vi "FPGA_8a_ws_BIdireccional.vi"() -> ()   [LabVIEW 2015]
doc: "This VI reads a buffer of single point values from all four channels of the NI 923x and places the acquired data into a DMA FIFO."
uses:
  <vilib>/LabVIEW Targets/FPGA/cRIO/shared/nicrio_ModuleControls/nicrio_cRIO-9234_DataRatesRing2.ctl
  <vilib>/LabVIEW Targets/FPGA/cRIO/shared/nicrio_ModuleControls/nicrio_BasicConversionTime.ctl
  <vilib>/rvi/Emulation/niFpgaGetClockAttributes.vi
  <vilib>/rvi/Emulation/niFpgaSctlEmulationGetInTimedLoop.vi
  <vilib>/rvi/Emulation/niFpgaEmulationReportErrorSimple.vi
  <vilib>/rvi/eio/common/nirviEmuTemplateMethod_errors.vi
  <vilib>/rvi/Emulation/niFpgaCriticalErrorInLSC.vi
  <vilib>/rvi/eio/common/nirviEmuTemplatePropertySet_errors.vi
  <vilib>/rvi/Emulation/niFpgaProcessEmulError.vi
  <vilib>/rvi/interface/RandomDataEmulation/niFpgaRandomDataHandleErrors.vi
  <vilib>/eio/EIONode/EIONode.xnode
  <vilib>/eio/EIOPropertyNode/EIOPropertyNode.xnode
  <vilib>/rvi/DataTransferAndStorage/Container/XNode/niFpgaContainer.xnode
  <vilib>/rvi/interface/RandomDataEmulation/nirviRandomDataFpgaReadWriteTemplate.vi
  <vilib>/rvi/eio/common/nirviEmuTemplatePropertyGet_errors.vi
  <vilib>/rvi/eio/common/nirviEmuTemplatePropertyGet_noerrors.vi
  <vilib>/rvi/eio/common/nirviEmuTemplatePropertySet_noerrors.vi
panel:
  out "Direccion 0?":bool
  in  "Digital?":bool=TRUE
  out "Numeric 2":i32
  out "WhlCnt":fxp<+/-,24,-4> format="%.27g"
  in  "Offset_rueda":fxp<+/-,24,-4> format="%.27g"
  out "Rueda?":i16
  in  "Conversion Time":T1
  in  "Canal ccero?":bool=TRUE
  in  "Count(mSec)":u32=2
  out "Chassis Temperature":i16
  out "Fotocelula":bool
  out "Detector de\npresencia":bool
  in  "Fotocélula":bool
  out "DC OK":bool
  in  "Data Rate":T2=2 items=["51.200 kS/s (NI 9234)"=1, "25.600 kS/s (NI 9234)"=2, "17.067 kS/s (NI 9234)"=3, "12.800 kS/s (NI 9234)"=4, "10.240 kS/s (NI 9234)"=5, "8.533 kS/s (NI 9234)"=6, "7.314 kS/s (NI 9234)"=7, "6.400 kS/s (NI 9234)"=8, "5.689 kS/s (NI 9234)"=9, "5.120 kS/s (NI 9234)"=10, "4.654 kS/s (NI 9234)"=11, "4.267 kS/s (NI 9234)"=12, "3.938 kS/s (NI 9234)"=13, "3.657 kS/s (NI 9234)"=14, "3.413 kS/s (NI 9234)"=15, "3.200 kS/s (NI 9234)"=16, "3.012 kS/s (NI 9234)"=17, "2.845 kS/s (NI 9234)"=18, "2.695 kS/s (NI 9234)"=19, "2.560 kS/s (NI 9234)"=20, "2.438 kS/s (NI 9234)"=21, "2.328 kS/s (NI 9234)"=22, "2.226 kS/s (NI 9234)"=23, "2.133 kS/s (NI 9234)"=24, "2.048 kS/s (NI 9234)"=25, "1.969 kS/s (NI 9234)"=26, "1.896 kS/s (NI 9234)"=27, "1.829 kS/s (NI 9234)"=28, "1.765 kS/s (NI 9234)"=29, "1.707 kS/s (NI 9234)"=30, "1.652 kS/s (NI 9234)"=31]
  out "Buffer Overflow":bool
  in  "Stop":bool
  out "Buffer Underflow":bool
  out "Error Out":errorcluster
  # "For instructions, and select Help>>Show Context Help and hover over the icon."
  # "Timing Parameters"
  # "Output Parameters"
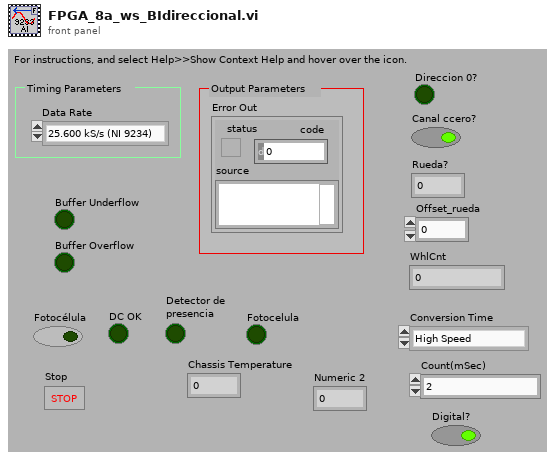
[diagram p1: front panel]
types:
  T1 = typedef "nicrio_BasicConversionTime.ctl" = enum8{"High Speed", "High Resolution"}
  T2 = typedef "nicrio_cRIO-9234_DataRatesRing2.ctl" = u8
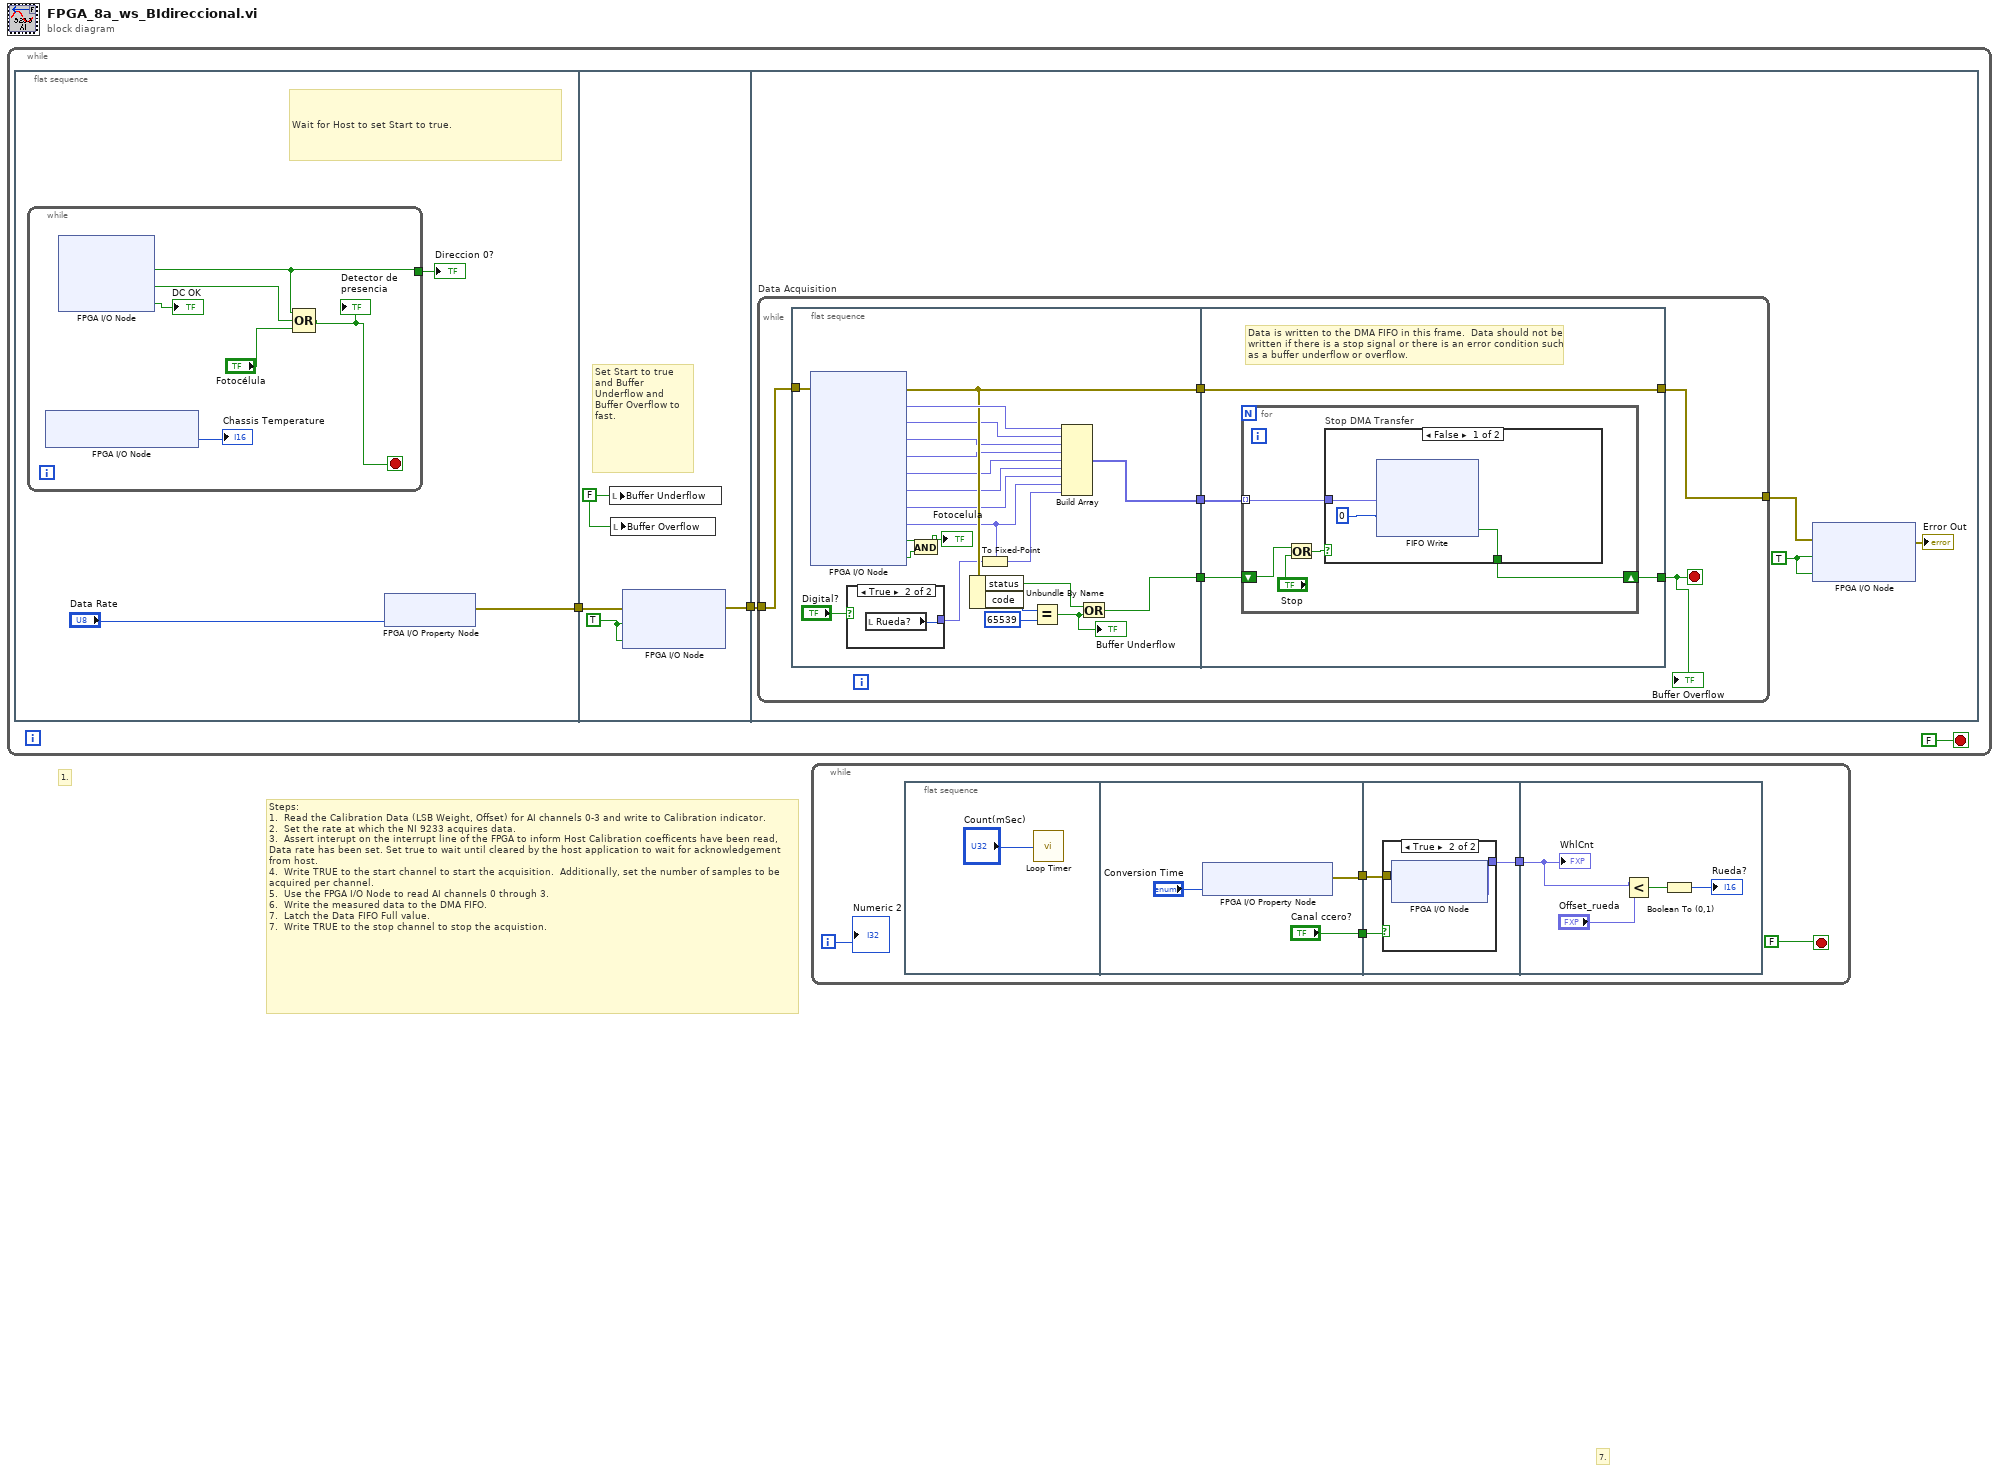
[diagram p0: block diagram]
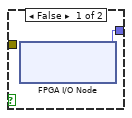
[diagram p2: hidden frame]
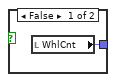
[diagram p3: hidden frame]
diagram:
  # "7."
  # "Steps: \n1.  Read the Calibration Data (LSB Weight, Offset) for AI channels 0-3 and write to Calibration indicator.\n2.  Set the rate at which the NI 9233 acquires data. \n3.  Assert interupt on the interrupt line of the FPGA to inform Host Calibration coefficents have been read, Data rate has been set. Set true to wait until cleared by the host application to wait for acknowledgement from host.\n4.  Write TRUE to the start channel to start the acquisition.  Additionally, set the number of samples to be acquired per channel.\n5.  Use the FPGA I/O Node to read AI channels 0 through 3. \n6.  Write the measured data to the DMA FIFO.\n7.  Latch the Data FIFO Full value.\n7.  Write TRUE to the stop channel to stop the acquistion."
  # "1."
  n1 = while {
    stop <- FALSE stop-if-true
    n2 = flat-sequence "MainSeq" {
      tunnel: [w6] -> w2
      tunnel: w2 -> [w15]
      tunnel: [w14] -> w1
      tunnel: w1 -> [w20]
      frame #0 {
        # "Wait for Host to set Start to true."
        n3 = while "initWait" {
          tunnel: [w7] -> w4
          stop <- w8 stop-if-true
          n4 = xnode "FPGA I/O Node"() -> ("Chassis Temperature"=→"Chassis Temperature":i16)  [unwired: 1 in, 1 out]
          n5 = xnode "FPGA I/O Node"() -> ("Mod3/DI0"=w7:bool, "Mod3/DI1"=w10:bool, "Mod3/DI2"=→"DC OK":bool)  [unwired: 4 in, 4 out]
          n6 = Compound Arithmetic op=OR(w7, w10, "Fotocélula") -> (w8:bool)
          "Detector de\npresencia" <- w8
        }
        "Direccion 0?" <- w4
        n7 = xnode "FPGA I/O Property Node"("Data Rate"="Data Rate") -> ("error out"=w6:errorcluster)  [unwired: 2 in, 1 out]
      }
      frame #1 {
        w13 = TRUE
        w16 = FALSE ("Late? (Latched)")
        # "Set Start to true and Buffer Underflow and Buffer Overflow to fast."
        n8 = local write "Buffer Underflow"(w16) -> ()
        n9 = local write "Buffer Overflow"(w16) -> ()
        n10 = xnode "FPGA I/O Node"("error in"=w15, "Mod1/Start"=w13, "Mod2/Start"=w13) -> ("error out"=w14:errorcluster)  [unwired: 2 in, 2 out]
      }
      frame #2 {
        w17 = TRUE
        n11 = while "Data Acquisition" {
          tunnel: w20 -> [w24]
          tunnel: [w23] -> w18
          stop <- w21 stop-if-true
          n12 = flat-sequence "Data Acquisition Sequence" {
            tunnel: [w47] -> w26
            tunnel: [w38] -> w25
            tunnel: w24 -> [w46]
            tunnel: [w45] -> w22
            tunnel: w26 -> [w54]
            tunnel: w25 -> [w53]
            tunnel: [w52] -> w21
            tunnel: [w51] -> w23
            tunnel: w22 -> [w51]
            frame #0 {
              n13 = xnode "FPGA I/O Node"("error in"=w46) -> ("error out"=w45:errorcluster, "Mod1/AI0"=w48:fxp<+/-,24,4>, "Mod1/AI1"=w41:fxp<+/-,24,4>, "Mod1/AI2"=w40:fxp<+/-,24,4>, "Mod1/AI3"=w39:fxp<+/-,24,4>, "Mod2/AI0"=w36:fxp<+/-,24,4>, "Mod2/AI1"=w35:fxp<+/-,24,4>, "Mod2/AI2"=w34:fxp<+/-,24,4>, "Mod2/AI3"=w33:fxp<+/-,24,4>, "Mod3/DI0"=w29:bool, "Mod3/DI1"=w28:bool)  [unwired: 10 in, 10 out]
              n14 = case shown="True" "Digital?" {
                tunnel: [w49 w50] -> w30
                frame False {
                  n15 = local read "WhlCnt"() -> (w49:fxp<+/-,24,-4>)
                }
                frame True {
                  n16 = local read "Rueda?"() -> (w50:i16)
                }
              }
              n17 = And(x=w29, y=w28) -> (x .and. y?=→"Fotocelula":bool)
              n18 = Unbundle By Name(w45) -> ("status"=w37:bool, "code"=w44:i32)
              n19 = To Fixed-Point(fixed-point type=w33, number=w30) -> (fixed-point=w32:fxp<+/-,24,4>)
              n20 = Equal?(x=w44, y=65539) -> (x = y?=w42:bool)
              "Buffer Underflow" <- w42
              n21 = Build Array(w48, w41, w40, w39, w36, w35, w34, w33, w32) -> (w47:fxp<+/-,24,4>[])
              n22 = Or(x=w37, y=w42) -> (x .or. y?=w38:bool)
            }
            frame #1 {
              # "Data is written to the DMA FIFO in this frame.  Data should not be\nwritten if there is a stop signal or there is an error condition such \nas a buffer underflow or overflow."
              n23 = for "DMAWriteLoop" {
                tunnel: w54 -> [w59] mode=indexing
                shift-right: [w55] -> w52
                shift-left: w53 -> [w57]
                n24 = Or(x=w57, y="Stop") -> (x .or. y?=w56:bool)
                n25 = case "Stop DMA Transfer" shown="False" w56 {
                  selector: w56 -> [_ w63]
                  tunnel: w59 -> [w60 _]
                  tunnel: [w62 w63] -> w55
                  frame False {
                    n26 = xnode ("FIFO Write")("Element"=w60, "Timeout"=0) -> ("Timed Out?"=w62:bool)  [unwired: 1 in, 1 out]
                  }
                  frame True {
                  }
                }
              }
            }
          }
          "Buffer Overflow" <- w21
        }
        n27 = xnode "FPGA I/O Node"("error in"=w18, "Mod1/Stop"=w17, "Mod2/Stop"=w17) -> ("error out"=→"Error Out":errorcluster)  [unwired: 2 in, 2 out]
      }
    }
  }
  n28 = while {
    i -> [w68]
    stop <- FALSE stop-if-true
    n29 = flat-sequence {
      tunnel: [w71] -> w66
      tunnel: ["Canal ccero?"] -> w64
      tunnel: [w75] -> w67
      tunnel: w66 -> [w74]
      tunnel: w64 -> [w73]
      tunnel: w67 -> [w81]
      frame #0 {
        n30 = call "Loop Timer"("Count(mSec)"="Count(mSec)") -> ()  [unwired: 1 out]
      }
      frame #1 {
        n31 = xnode "FPGA I/O Property Node"("Conversion Time"="Conversion Time") -> ("error out"=w71:errorcluster)  [unwired: 2 in, 1 out]
      }
      frame #2 {
        n32 = case shown="True" w73 {
          tunnel: [w76 w78] -> w75
          tunnel: w74 -> [_ w77]
          frame False {
            n33 = xnode "FPGA I/O Node"() -> ("Mod4/AI1"=w76:fxp<+/-,24,-4>)  [unwired: 2 in, 2 out]
          }
          frame True {
            n34 = xnode "FPGA I/O Node"("error in"=w77) -> ("Mod4/AI0"=w78:fxp<+/-,24,-4>)  [unwired: 1 in, 2 out]
          }
        }
      }
      frame #3 {
        n35 = Less?(x=w81, y="Offset_rueda") -> (x < y?=w80:bool)
        n36 = Boolean To (0,1)(Boolean=w80) -> (0, 1=→"Rueda?":i16)
        "WhlCnt" <- w81
      }
    }
    "Numeric 2" <- w68
  }
